vi "AUTON_Index.vi"(0 "Auton Array":dbl[][](array[numeric]), 5 "MeasuredHeading":dbl, 7 "LeftEncoder":dbl, 9 "RightEncoder":dbl) -> (4 "Right Drive":dbl, 6 "Left Drive":dbl, 8 "Harvester":dbl, 10 "Winch":dbl, 14 "Roller":dbl, 15 "Cam":dbl)   [LabVIEW 2013]
uses:
  Robot Global Data.vi
panel:
  out "AT4":bool
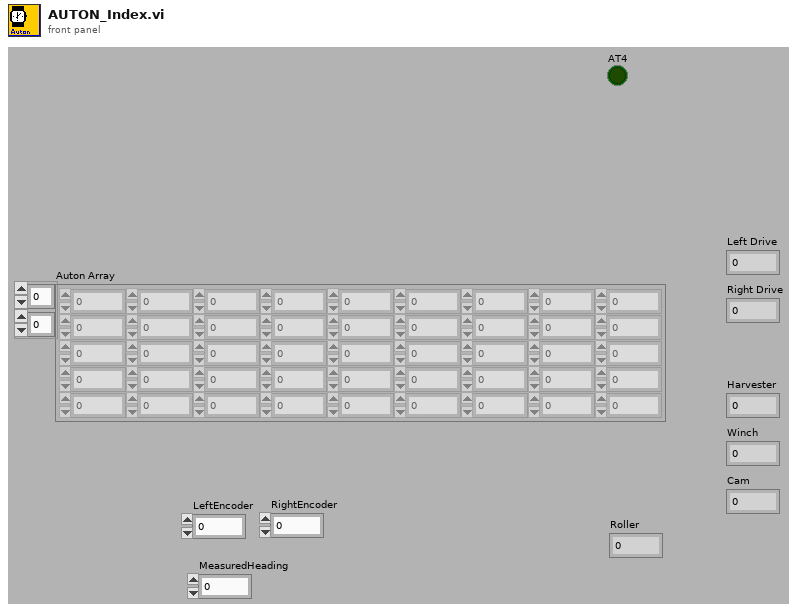
[diagram p1: front panel]
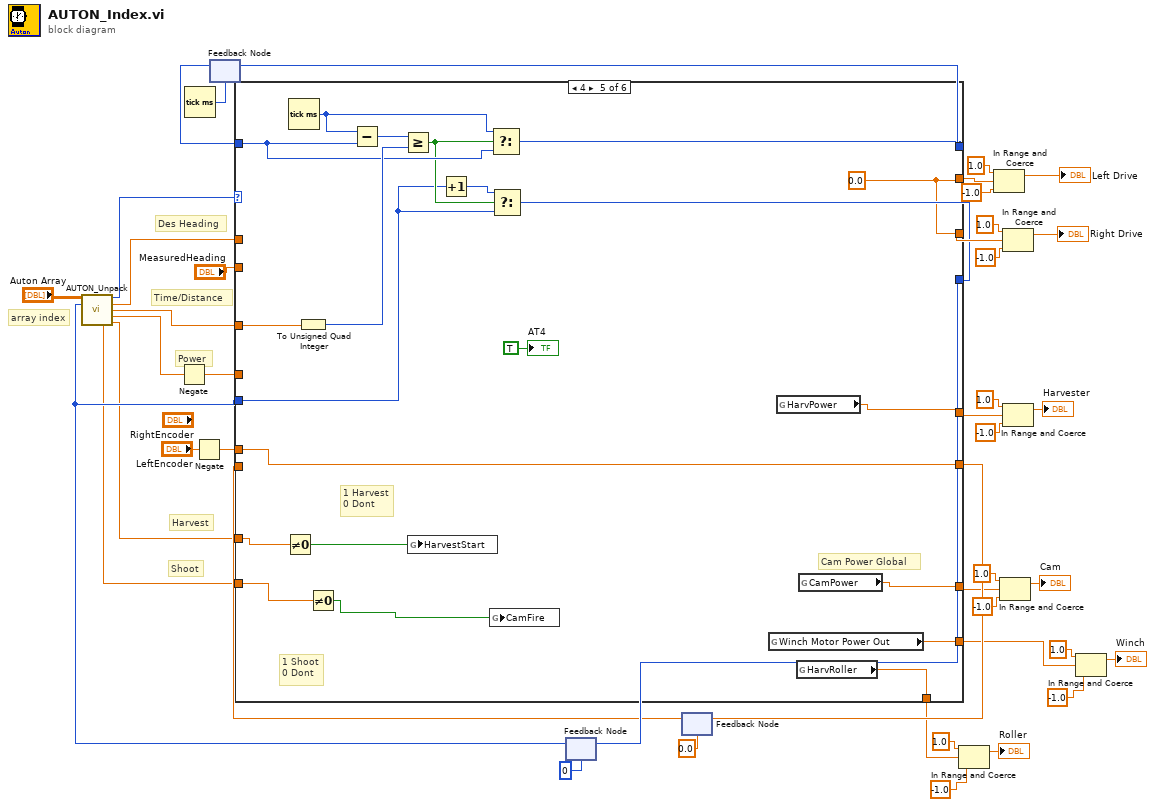
[diagram p0: block diagram]
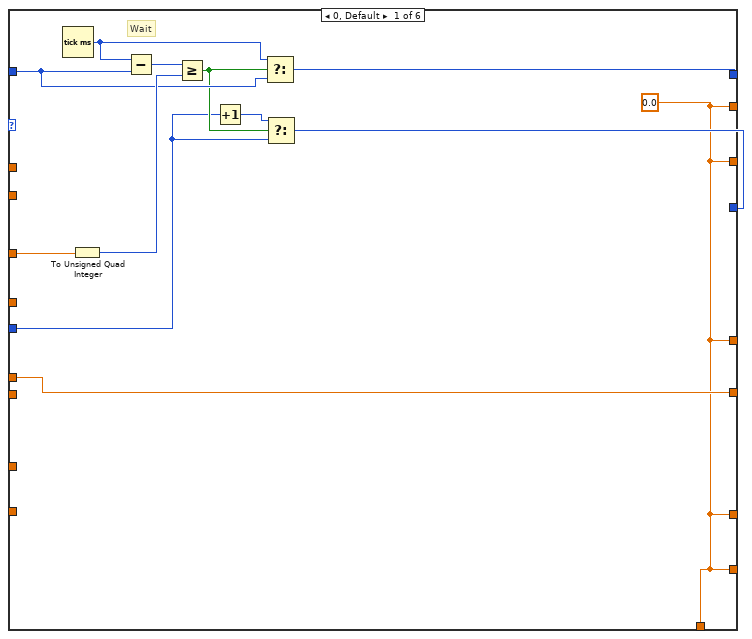
[diagram p2: hidden frame]
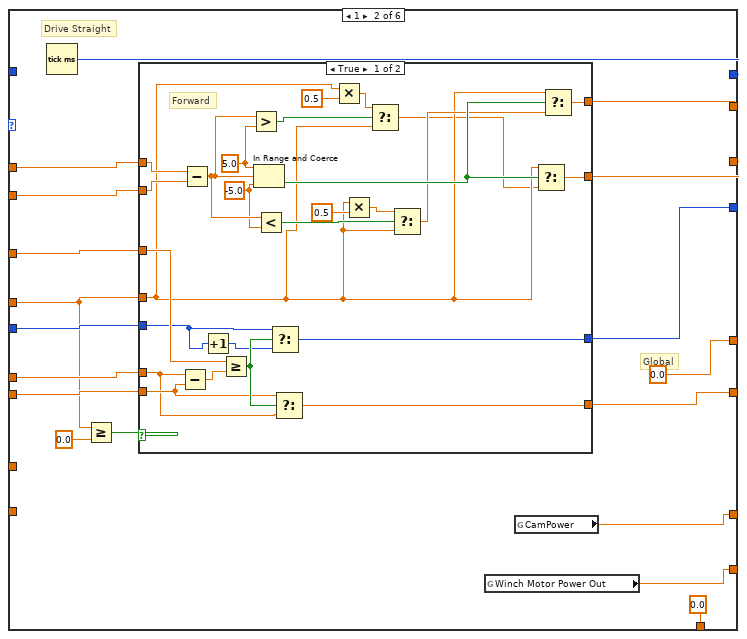
[diagram p3: hidden frame]
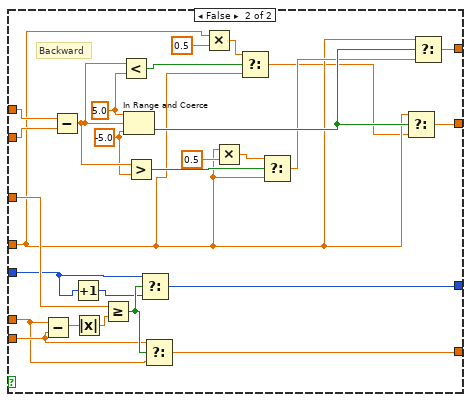
[diagram p4: hidden frame]
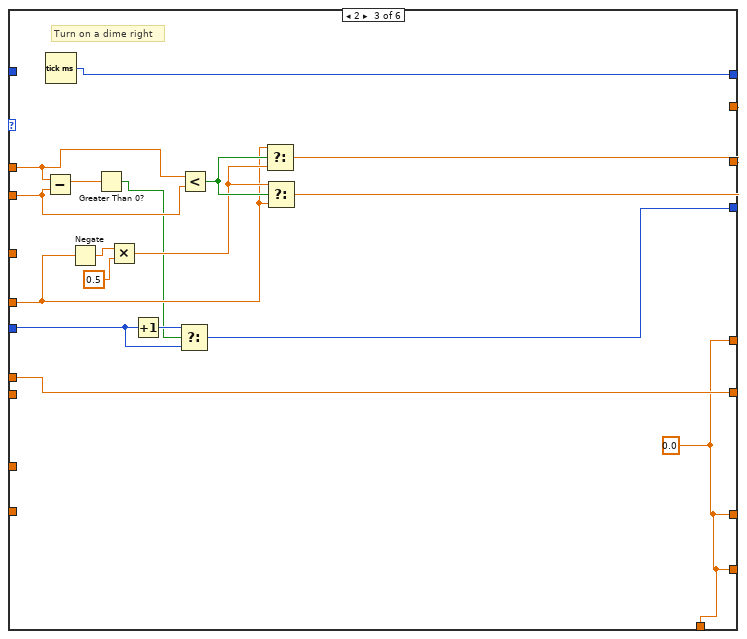
[diagram p5: hidden frame]
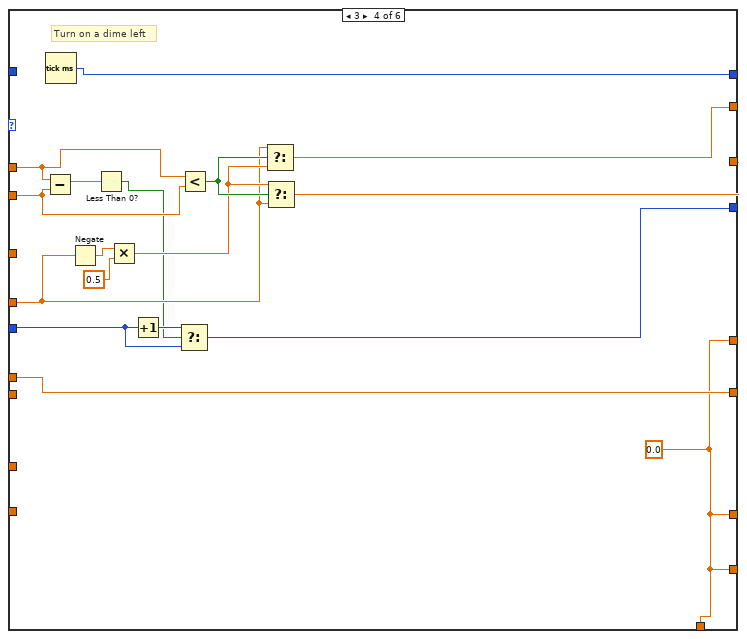
[diagram p6: hidden frame]
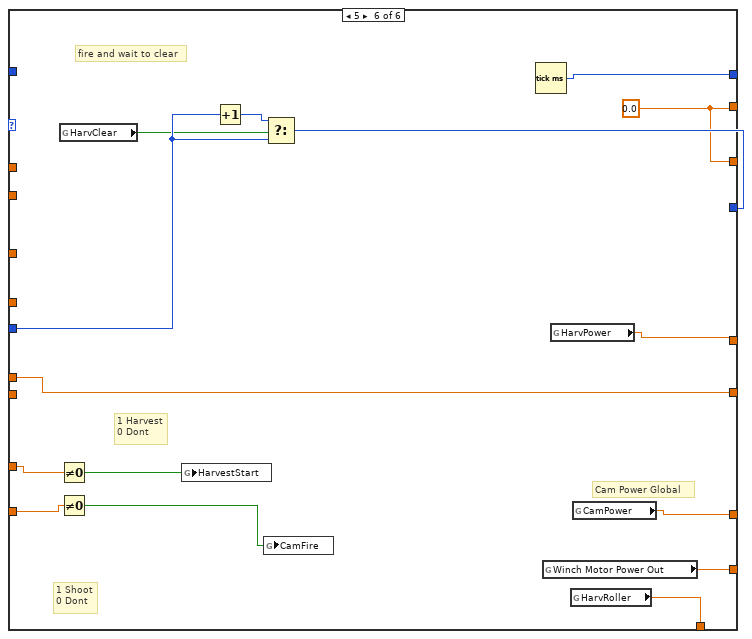
[diagram p7: hidden frame]
diagram:
  # "Shoot"
  # "Harvest"
  # "Des Heading"
  # "Time/Distance"
  # "Power"
  # "array index"
  n1 = Tick Count (ms)() -> (millisecond timer value=w42:u32)
  n2 = Negate(x="LeftEncoder") -> (-x=w8:dbl)
  n3 = feedback #1(w42) -> (w43:u32)
  n4 = feedback #2(0) -> (w23:i32)
  n5 = call "AUTON_Unpack.vi"("all rows"="Auton Array", "Index"=w23) -> ("Primitive ID"=w26:i16, "Desired Heading"=w25:dbl, "Time/Distance"=w24:dbl, "Power"=w11:dbl, "Shoot"=w6:dbl, "Harvest"=w7:dbl)  [unwired: 8 in]
  n6 = Negate(x=w11) -> (-x=w10:dbl)
  n7 = feedback #3(0.0) -> (w28:dbl)
  n8 = case shown="4" w26 {
    tunnel: [w48 w72 w139 w156 w174 w195] -> w30
    tunnel: w23 -> [w49 w67 w142 w159 w175 w196]
    tunnel: [w56 w64 w144 w161 w182 w186] -> w32
    tunnel: w43 -> [w53 _ _ _ w179 _]
    tunnel: w24 -> [w47 w73 _ _ w173 _]
    tunnel: w25 -> [_ w71 w137 w154 _ _]
    tunnel: [w45 w69 w140 w157 w172 w194] -> w40
    tunnel: [w45 w68 w141 w158 w172 w194] -> w33
    tunnel: w10 -> [_ w63 w131 w148 _ _]
    tunnel: w8 -> [w46 w65 w138 w155 w171 w193]
    tunnel: "MeasuredHeading" -> [_ w70 w136 w153 _ _]
    tunnel: w28 -> [_ w66 _ _ _ _]
    tunnel: [w46 w74 w138 w155 w171 w193] -> w27
    tunnel: [w45 w59 w128 w145 w169 w191] -> w13
    tunnel: [w45 0.0 ("OutWheelF") w128 w145 w170 w192] -> w12
    tunnel: w7 -> [_ _ _ _ w166 w189]
    tunnel: w6 -> [_ _ _ _ w168 w184]
    tunnel: [w45 w58 w128 w145 w167 w190] -> w5
    tunnel: [w45 0.0 ("HarvRoller") w128 w145 w163 w187] -> w1
    frame 0, Default {
      w45 = 0.0 ("Numeric")
      # "Wait"
      n9 = Tick Count (ms)() -> (millisecond timer value=w52:u32)
      n10 = To Unsigned Quad Integer(1:w47) -> (0:w54:u64)
      n11 = Subtract(x=w52, y=w53) -> (x-y=w55:u32)
      n12 = Greater Or Equal?(x=w55, y=w54) -> (x >= y?=w51:bool)
      n13 = Increment(x=w49) -> (x+1=w50:i32)
      n14 = Select(t=w52, s=w51, f=w53) -> (s? t:f=w56:u32)
      n15 = Select(t=w50, s=w51, f=w49) -> (s? t:f=w48:i32)
    }
    frame 1 {
      # "Global"
      # "Drive Straight"
      n16 = Tick Count (ms)() -> (millisecond timer value=w64:u32)
      n17 = Greater Or Equal?(x=w63, y=0.0) -> (x >= y?=w61:bool)
      n18 = case shown="True" w61 {
        tunnel: [w100 w127] -> w74
        tunnel: w73 -> [w98 w126]
        tunnel: [w96 w124] -> w72
        tunnel: w71 -> [w95 w123]
        tunnel: w70 -> [w94 w122]
        tunnel: [w92 w120] -> w69
        tunnel: [w91 w119] -> w68
        tunnel: w63 -> [w80 w108]
        tunnel: w67 -> [w77 w105]
        tunnel: w66 -> [w76 w104]
        tunnel: w65 -> [w75 w103]
        frame True {
          w88 = -5.0 ("lower limit")
          w90 = 5.0 ("upper limit")
          # "Forward"
          n19 = Subtract(x=w75, y=w76) -> (x-y=w99:dbl)
          n20 = Subtract(x=w95, y=w94) -> (x-y=w89:dbl)
          n21 = Increment(x=w77) -> (x+1=w78:i32)
          n22 = Greater Or Equal?(x=w98, y=w99) -> (x >= y?=w97:bool)
          n23 = Greater?(x=w89, y=w90) -> (0:w83:bool)
          n24 = In Range and Coerce(upper limit=w90, x=w89, lower limit=w88) -> (In Range?=w93:bool)  [unwired: 1 out]
          n25 = Less?(x=w89, y=w88) -> (x < y?=w87:bool)
          n26 = Select(t=w77, s=w97, f=w78) -> (s? t:f=w96:i32)
          n27 = Select(t=w76, s=w97, f=w75) -> (s? t:f=w100:dbl)
          n28 = Multiply(x=w80, y=0.5) -> (x*y=w82:dbl)
          n29 = Multiply(x=w80, y=0.5) -> (x*y=w85:dbl)
          n30 = Select(t=w82, s=w83, f=w80) -> (s? t:f=w79:dbl)
          n31 = Select(t=w85, s=w87, f=w80) -> (s? t:f=w84:dbl)
          n32 = Select(t=w80, s=w93, f=w79) -> (s? t:f=w91:dbl)
          n33 = Select(t=w80, s=w93, f=w84) -> (s? t:f=w92:dbl)
        }
        frame False {
          w116 = -5.0 ("lower limit")
          w118 = 5.0 ("upper limit")
          # "Backward"
          n34 = Subtract(x=w103, y=w104) -> (x-y=w101:dbl)
          n35 = Subtract(x=w123, y=w122) -> (x-y=w117:dbl)
          n36 = Increment(x=w105) -> (x+1=w106:i32)
          n37 = Absolute Value(x=w101) -> (abs(x)=w102:dbl)
          n38 = Greater Or Equal?(x=w126, y=w102) -> (x >= y?=w125:bool)
          n39 = Less?(x=w117, y=w118) -> (x < y?=w111:bool)
          n40 = In Range and Coerce(upper limit=w118, x=w117, lower limit=w116) -> (In Range?=w121:bool)  [unwired: 1 out]
          n41 = Greater?(x=w117, y=w116) -> (0:w115:bool)
          n42 = Select(t=w105, s=w125, f=w106) -> (s? t:f=w124:i32)
          n43 = Select(t=w104, s=w125, f=w103) -> (s? t:f=w127:dbl)
          n44 = Multiply(x=w108, y=0.5) -> (x*y=w110:dbl)
          n45 = Multiply(x=w108, y=0.5) -> (x*y=w113:dbl)
          n46 = Select(t=w110, s=w111, f=w108) -> (s? t:f=w107:dbl)
          n47 = Select(t=w113, s=w115, f=w108) -> (s? t:f=w112:dbl)
          n48 = Select(t=w108, s=w121, f=w107) -> (s? t:f=w119:dbl)
          n49 = Select(t=w108, s=w121, f=w112) -> (s? t:f=w120:dbl)
        }
      }
      n50 = global read "Robot Global Data.vi" "Winch Motor Power Out"() -> (w58:dbl)
      n51 = global read "Robot Global Data.vi" "CamPower"() -> (w59:dbl)
    }
    frame 2 {
      w128 = 0.0 ("Numeric")
      # "Turn on a dime right"
      n52 = Subtract(x=w137, y=w136) -> (x-y=w130:dbl)
      n53 = Tick Count (ms)() -> (millisecond timer value=w144:u32)
      n54 = Negate(x=w131) -> (-x=w134:dbl)
      n55 = Greater Than 0?(x=w130) -> (x > 0?=w129:bool)
      n56 = Multiply(x=w134, y=0.5) -> (x*y=w132:dbl)
      n57 = Increment(x=w142) -> (x+1=w143:i32)
      n58 = Select(t=w143, s=w129, f=w142) -> (s? t:f=w139:i32)
      n59 = Less?(x=w137, y=w136) -> (x < y?=w135:bool)
      n60 = Select(t=w131, s=w135, f=w132) -> (s? t:f=w140:dbl)
      n61 = Select(t=w132, s=w135, f=w131) -> (s? t:f=w141:dbl)
    }
    frame 3 {
      w145 = 0.0 ("Numeric")
      # "Turn on a dime left"
      n62 = Subtract(x=w154, y=w153) -> (x-y=w147:dbl)
      n63 = Tick Count (ms)() -> (millisecond timer value=w161:u32)
      n64 = Negate(x=w148) -> (-x=w151:dbl)
      n65 = Less Than 0?(x=w147) -> (x < 0?=w146:bool)
      n66 = Multiply(x=w151, y=0.5) -> (x*y=w149:dbl)
      n67 = Increment(x=w159) -> (x+1=w160:i32)
      n68 = Select(t=w160, s=w146, f=w159) -> (s? t:f=w156:i32)
      n69 = Less?(x=w154, y=w153) -> (x < y?=w152:bool)
      n70 = Select(t=w148, s=w152, f=w149) -> (s? t:f=w157:dbl)
      n71 = Select(t=w149, s=w152, f=w148) -> (s? t:f=w158:dbl)
    }
    frame 4 {
      w172 = 0.0 ("Numeric")
      # "1 Harvest\n0 Dont"
      # "1 Shoot\n0 Dont"
      # "Cam Power Global"
      n72 = Not Equal To 0?(x=w166) -> (x != 0?=w165:bool)
      n73 = Tick Count (ms)() -> (millisecond timer value=w178:u32)
      n74 = To Unsigned Quad Integer(1:w173) -> (0:w180:u64)
      n75 = Not Equal To 0?(x=w168) -> (x != 0?=w164:bool)
      n76 = Subtract(x=w178, y=w179) -> (x-y=w181:u32)
      n77 = Greater Or Equal?(x=w181, y=w180) -> (x >= y?=w177:bool)
      n78 = global write "Robot Global Data.vi" "HarvestStart"(w165) -> ()
      n79 = Increment(x=w175) -> (x+1=w176:i32)
      n80 = global write "Robot Global Data.vi" "CamFire"(w164) -> ()
      n81 = Select(t=w178, s=w177, f=w179) -> (s? t:f=w182:u32)
      n82 = Select(t=w176, s=w177, f=w175) -> (s? t:f=w174:i32)
      n83 = global read "Robot Global Data.vi" "Winch Motor Power Out"() -> (w167:dbl)
      n84 = global read "Robot Global Data.vi" "HarvPower"() -> (w170:dbl)
      n85 = global read "Robot Global Data.vi" "HarvRoller"() -> (w163:dbl)
      n86 = global read "Robot Global Data.vi" "CamPower"() -> (w169:dbl)
      "AT4" <- TRUE ("x >= y?")
    }
    frame 5 {
      w194 = 0.0 ("Numeric")
      # "fire and wait to clear"
      # "1 Harvest\n0 Dont"
      # "1 Shoot\n0 Dont"
      # "Cam Power Global"
      n87 = Not Equal To 0?(x=w189) -> (x != 0?=w188:bool)
      n88 = Not Equal To 0?(x=w184) -> (x != 0?=w183:bool)
      n89 = global read "Robot Global Data.vi" "HarvClear"() -> (w185:bool)
      n90 = global write "Robot Global Data.vi" "HarvestStart"(w188) -> ()
      n91 = Increment(x=w196) -> (x+1=w197:i32)
      n92 = global write "Robot Global Data.vi" "CamFire"(w183) -> ()
      n93 = Select(t=w197, s=w185, f=w196) -> (s? t:f=w195:i32)
      n94 = Tick Count (ms)() -> (millisecond timer value=w186:u32)
      n95 = global read "Robot Global Data.vi" "Winch Motor Power Out"() -> (w190:dbl)
      n96 = global read "Robot Global Data.vi" "HarvPower"() -> (w192:dbl)
      n97 = global read "Robot Global Data.vi" "HarvRoller"() -> (w187:dbl)
      n98 = global read "Robot Global Data.vi" "CamPower"() -> (w191:dbl)
    }
  }
  n99 = feedback-in #1(w32) -> ()
  n100 = feedback-in #2(w30) -> ()
  n101 = feedback-in #3(w27) -> ()
  n102 = In Range and Coerce(upper limit=1.0, x=w1, lower limit=-1.0) -> (coerced(x)=→"Roller":dbl)  [unwired: 1 out]
  n103 = In Range and Coerce(upper limit=1.0, x=w40, lower limit=-1.0) -> (coerced(x)=→"Left Drive":dbl)  [unwired: 1 out]
  n104 = In Range and Coerce(upper limit=1.0, x=w13, lower limit=-1.0) -> (coerced(x)=→"Cam":dbl)  [unwired: 1 out]
  n105 = In Range and Coerce(upper limit=1.0, x=w33, lower limit=-1.0) -> (coerced(x)=→"Right Drive":dbl)  [unwired: 1 out]
  n106 = In Range and Coerce(upper limit=1.0, x=w12, lower limit=-1.0) -> (coerced(x)=→"Harvester":dbl)  [unwired: 1 out]
  n107 = In Range and Coerce(upper limit=1.0, x=w5, lower limit=-1.0) -> (coerced(x)=→"Winch":dbl)  [unwired: 1 out]
